vi "Breaker.vi"() -> ()   [LabVIEW 2019]
panel:
  in  "Heat Limit":dbl[unit]=1000000.0
  out "Current Supplied":dbl[unit]
  in  "Allowed Current":dbl[unit]=40.0
  out "Status":bool
  in  "Current Demand":dbl[unit](slide) scale=0.0..300.0
  out "Chart":T1(graph)
  in  "Breaker Characterization":T2
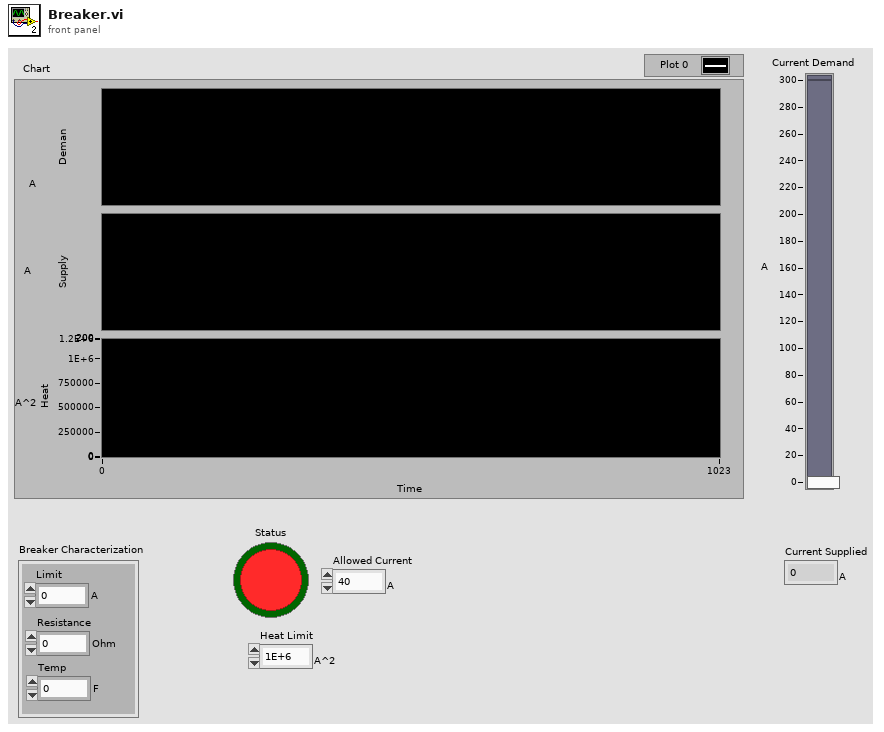
[diagram p1: front panel]
types:
  T1 = cluster{"Current Demand":dbl[unit], "Current Demand":dbl[unit], "lower limit":dbl[unit]}
  T2 = cluster{"Limit":dbl[unit], "Resistance":dbl[unit], "Temp":dbl[unit]}
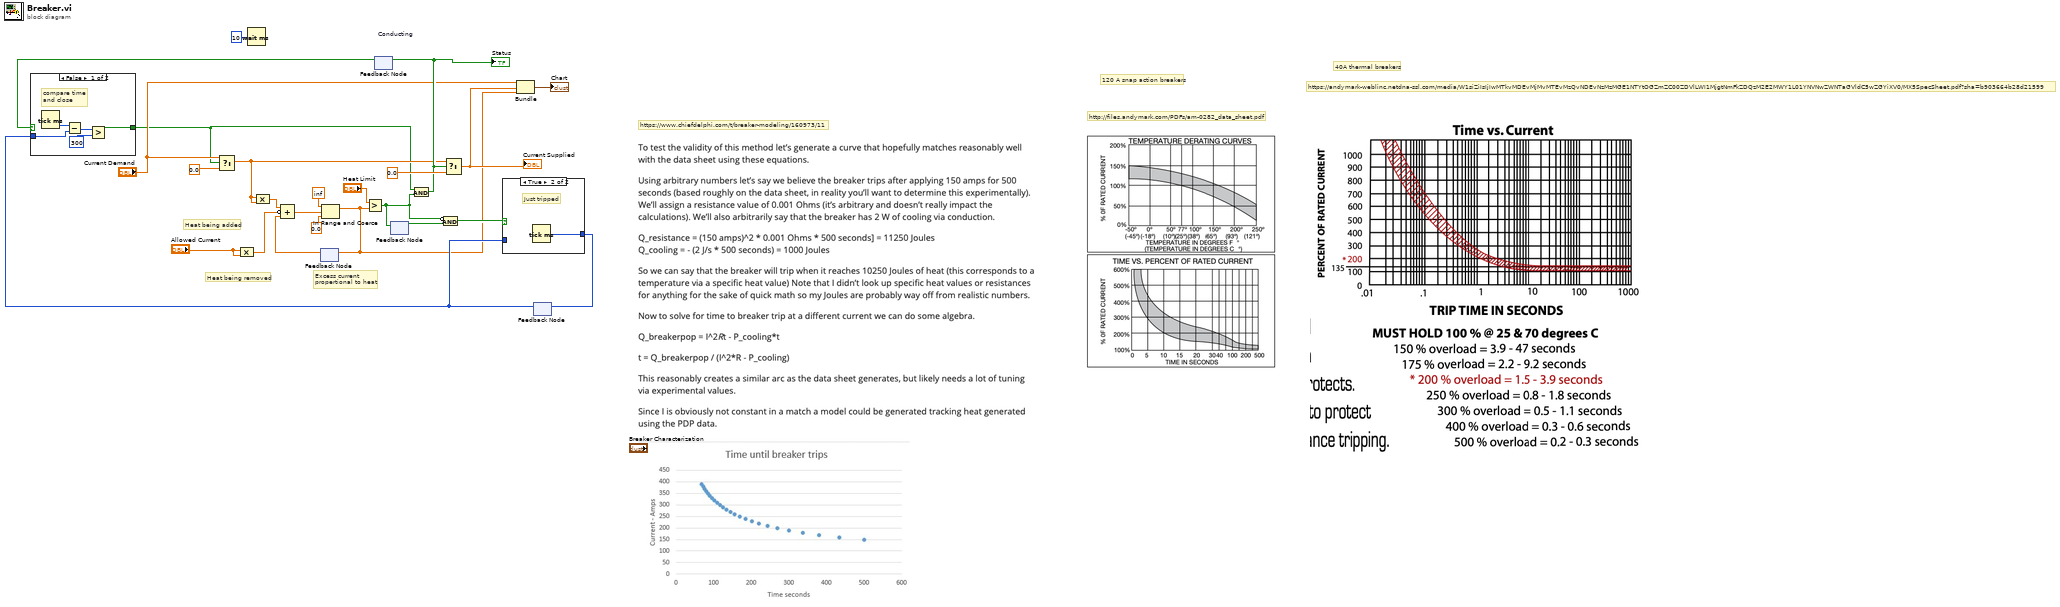
[diagram p0: block diagram]
diagram:
  # "Heat being added"
  # "Heat being removed"
  # "Excess current\npropertional to heat"
  # "40A thermal breakers"
  # "120 A snap action breakers"
  # "https://andymark-weblinc.netdna-ssl.com/media/W1siZiIsIjIwMTkvMDEvMjMvMTEvMzQvNDEvNzMzMGE1NTYtOGZmZC00ZDVlLWI1MjgtNmFkZDQzM2E2MWY1L01YNVNwZWNTaGVldC5wZGYiXV0/MX5SpecSheet.pdf?sha=b903664b28d21599"
  # "http://files.andymark.com/PDFs/am-0282_data_sheet.pdf"
  # "https://www.chiefdelphi.com/t/breaker-modeling/160973/11"
  n1 = Compound Arithmetic op=MULTIPLY("Allowed Current", "Allowed Current") -> (w22:dbl[unit])
  n2 = Wait (ms)(milliseconds to wait=u32 10) -> ()  [unwired: 1 out]
  n3 = feedback #1() -> (w24:dbl[unit])  [unwired: 1 in]
  n4 = feedback #2 "Conducting"() -> (w16:bool)  [unwired: 1 in]
  n5 = feedback #3() -> (w15:bool)  [unwired: 1 in]
  n6 = feedback #4() -> (w12:u32)  [unwired: 1 in]
  n7 = case shown="False" w16 {
    selector: w16 -> [_ w30]
    tunnel: [w25 w30] -> w1
    tunnel: w12 -> [w28 _]
    frame False {
      # "compare time\nand close"
      n8 = Tick Count (ms)() -> (millisecond timer value=w29:u32)
      n9 = Subtract(x=w29, y=w28) -> (x-y=w27:u32)
      n10 = Greater?(x=w27, y=300) -> (0:w25:bool)
    }
    frame True {
    }
  }
  n11 = Select(t="Current Demand", s=w1, f=dbl[unit] 0.0 ("Current Demand")) -> (s? t:f=w2:dbl[unit])
  n12 = Compound Arithmetic op=MULTIPLY(w2, w2) -> (w21:dbl[unit])
  n13 = Compound Arithmetic op=ADD(w21, invert w22, w24) -> (w18:dbl[unit])
  n14 = In Range and Coerce(upper limit=dbl[unit] inf, x=w18, lower limit=dbl[unit] 0.0) -> (coerced(x)=w10:dbl[unit])  [unwired: 1 out]
  n15 = feedback-in #1(w10) -> ()
  n16 = Greater?(x="Heat Limit", y=w10) -> (0:w6:bool)
  n17 = feedback-in #3(w6) -> ()
  n18 = Compound Arithmetic op=AND(w1, w6) -> (w5:bool)
  "Status" <- w5
  n19 = feedback-in #2(w5) -> ()
  n20 = Compound Arithmetic op=AND(invert w6, w15) -> (w14:bool)
  n21 = Select(t=w2, s=w5, f=dbl[unit] 0.0 ("Current Demand")) -> (s? t:f=w11:dbl[unit])
  "Current Supplied" <- w11
  n22 = case shown="True" w14 {
    tunnel: [w31 w32] -> w13
    tunnel: w12 -> [w31 _]
    frame False {
    }
    frame True {
      # "Just tripped"
      n23 = Tick Count (ms)() -> (millisecond timer value=w32:u32)
    }
  }
  n24 = Bundle("Current Demand"="Current Demand", "Current Demand"=w11, "lower limit"=w10) -> (→"Chart":T1)  [unwired: 1 in]
  n25 = feedback-in #4(w13) -> ()
